vi "UART Configure Parameters.vi"(0 "UART Driver in":refnum<class "UART Driver.lvclass">, 1 "Channel Number":u8, 5 "Baud":u32=4, 7 "Character Length":u8=8, 9 "Stop Bits":T1, 11 "error in":errorcluster, 12 "Parity":T2) -> (4 "UART Driver out":refnum<class "UART Driver.lvclass">, 15 "error out":errorcluster)   [LabVIEW 2012, in "UART_Host_Driver.lvlib" / "UART Driver.lvclass"]
uses:
  UART Driver.lvclass
  FPGA/UART/Parity.ctl
  FPGA/UART/StopBits.ctl
  FPGA/UART/UART_Firmware.lvlib
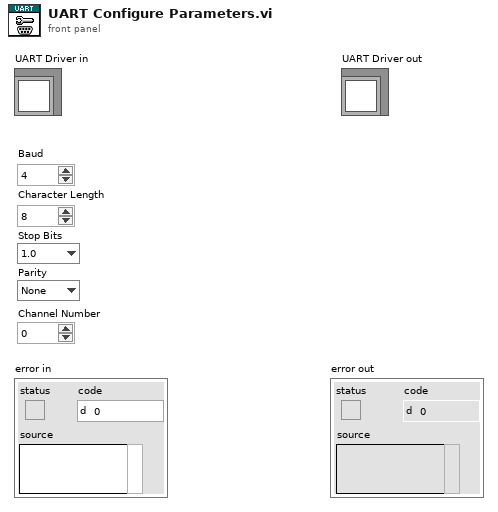
[diagram p1: front panel]
types:
  T1 = typedef "UART_Firmware.lvlib/StopBits.ctl" = enum8{"1.0", "1.5", "2.0"}
  T2 = typedef "UART_Firmware.lvlib/Parity.ctl" = enum8{"None", "Even", "Odd"}
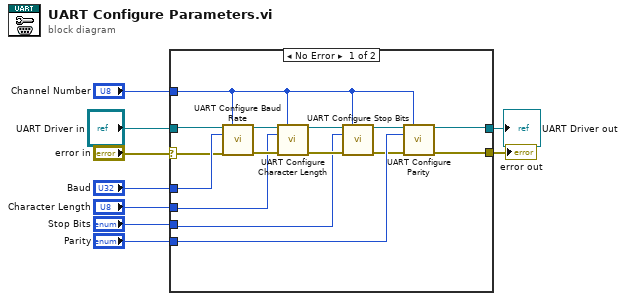
[diagram p0: block diagram]
diagram:
  n1 = case shown="No Error" "error in" {
    selector: "error in" -> [w22 w26]
    tunnel: [w11 w26] -> w8
    tunnel: [w10 w25] -> w1
    tunnel: "UART Driver in" -> [w24 w25]
    tunnel: "Baud" -> [w23 _]
    tunnel: "Character Length" -> [w19 _]
    tunnel: "Stop Bits" -> [w13 _]
    tunnel: "Parity" -> [w18 _]
    tunnel: "Channel Number" -> [w16 _]
    frame No Error {
      n2 = call-dynamic "UART Configure Baud Rate.vi"("UART Driver in"=w24, "Channel Number"=w16, "Baud Rate"=w23, "error in"=w22) -> ("UART Driver out"=w21:refnum<class "UART Driver.lvclass">, "error out"=w20:errorcluster)  [unwired: 9 in, 1 out]
      n3 = call-dynamic "UART Configure Character Length.vi"("UART Driver in"=w21, "Channel Number"=w16, "Character Length"=w19, "error in"=w20) -> ("UART Driver out"=w15:refnum<class "UART Driver.lvclass">, "error out"=w14:errorcluster)  [unwired: 9 in, 1 out]
      n4 = call-dynamic "UART Configure Stop Bits.vi"("UART Driver in"=w15, "Channel Number"=w16, "Stop Bits"=w13, "error in"=w14) -> ("UART Driver out"=w17:refnum<class "UART Driver.lvclass">, "error out"=w12:errorcluster)  [unwired: 9 in, 1 out]
      n5 = call-dynamic "UART Configure Parity.vi"("UART Driver in"=w17, "Channel Number"=w16, "Parity"=w18, "error in"=w12) -> ("UART Driver out"=w10:refnum<class "UART Driver.lvclass">, "error out"=w11:errorcluster)  [unwired: 9 in, 1 out]
    }
    frame Error {
    }
  }
  "error out" <- w8
  "UART Driver out" <- w1
